vi "Make Drink.vi"(8 "error in (no error)":errorcluster, 10 "Order Item in":refnum<class "Order Item.lvclass">, 11 "Barista in":refnum<class "Barista.lvclass">) -> (0 "error out":errorcluster, 2 "Order Item out":refnum<class "Order Item.lvclass">, 3 "Barista out":refnum<class "Barista.lvclass">)   [LabVIEW 2020, in "Barista.lvclass"]
uses:
  Barista.lvclass
  Support/Order Item/Order Item.lvclass
  Barista.lvclass/Barista.ctl
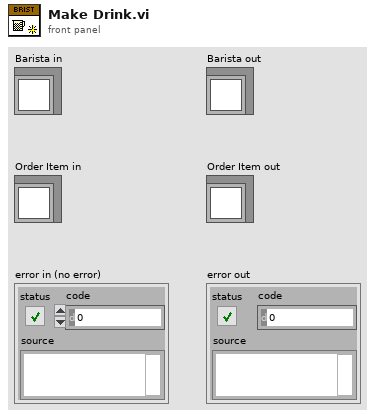
[diagram p1: front panel]
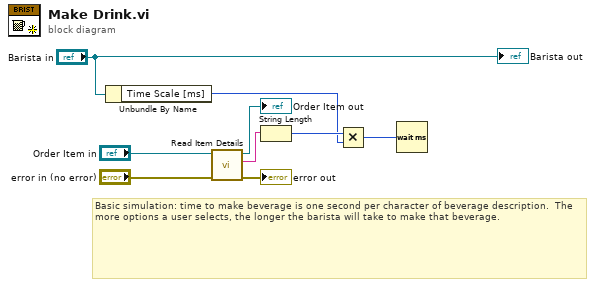
[diagram p0: block diagram]
diagram:
  # "Basic simulation: time to make beverage is one second per character of beverage description.  The more options a user selects, the longer the barista will take to make that beverage."
  n1 = Unbundle By Name("Barista in") -> ("Time Scale [ms]"=w1:u32)
  n2 = call-dynamic "Read Item Details.vi"("error in (no error)"="error in (no error)", "Order Item in"="Order Item in") -> ("error out"=→"error out":errorcluster, "Description"=w3:string, "Order Item out"=→"Order Item out":refnum<class "Order Item.lvclass">)  [unwired: 7 in]
  n3 = String Length(string=w3) -> (length=w5:i32)
  n4 = Multiply(x=w5, y=w1) -> (x*y=w4:u32)
  n5 = Wait (ms)(milliseconds to wait=w4) -> ()  [unwired: 1 out]
  "Barista out" <- "Barista in"
